vi "Zero Padded String.vi"(5 "Address (00)":i32 format="%0#2.0f") -> (6 "Zero Padded Address String":string)   [LabVIEW 2015]
doc: "This VI adds zeros the the beginning of a string as necessary to bring the string length to 2."
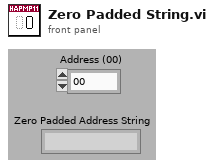
[diagram p1: front panel]
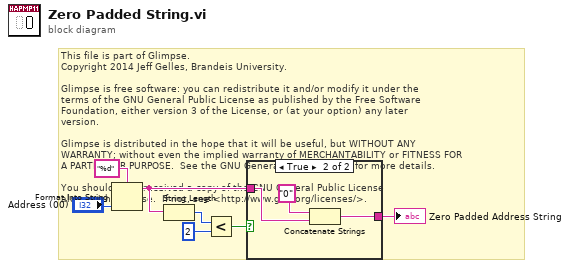
[diagram p0: block diagram]
diagram:
  # "This file is part of Glimpse. \nCopyright 2014 Jeff Gelles, Brandeis University.    \n\nGlimpse is free software: you can redistribute it and/or modify it under the \nterms of the GNU General Public License as published by the Free Software \nFoundation, either version 3 of the License, or (at your option) any later \nversion.\n\nGlimpse is distributed in the hope that it will be useful, but WITHOUT ANY \nWARRANTY; without even the implied warranty of MERCHANTABILITY or FITNESS FOR \nA PARTICULAR PURPOSE.  See the GNU General Public License for more details.\n\nYou should have received a copy of the GNU General Public License\nalong with Glimpse.  If not, see <http://www.gnu.org/licenses/>."
  n1 = Format Into String(format string="%d", "Address (00)") -> (resulting string=w1:string)  [unwired: 2 in, 1 out]
  n2 = String Length(string=w1) -> (length=w4:i32)
  n3 = Less?(x=w4, y=2) -> (x < y?=w6:bool)
  n4 = case shown="True" w6 {
    tunnel: [w8 w10] -> w5
    tunnel: w1 -> [w8 w9]
    frame False {
    }
    frame True {
      n5 = Concatenate Strings("0" ("string"), w9) -> (w10:string)
    }
  }
  "Zero Padded Address String" <- w5
